vi "Intan_writeDataAcqTimestamp.vi"(3 "hdr fpath":path) -> (1 "timestamp string":string)   [LabVIEW 2020]
panel:
  out "LabVIEW TimeStamp":timestamp
  out "Date Formatted with Milliseconds":string
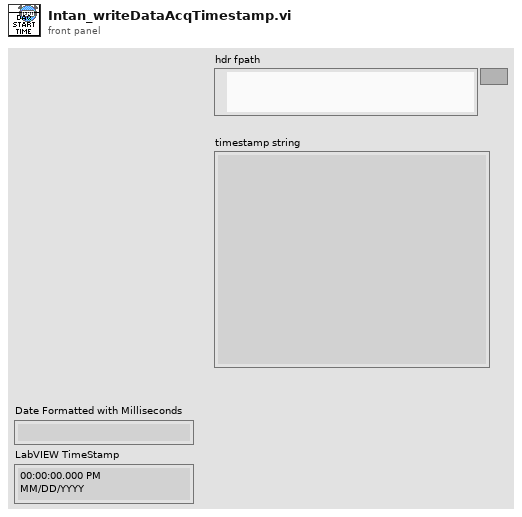
[diagram p1: front panel]
types:
  T1 = enum16{"open", "replace", "create", "open or create", "replace or create", "replace or create with confirmation"}
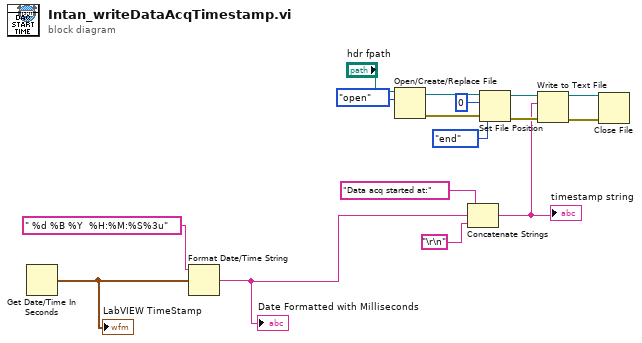
[diagram p0: block diagram]
diagram:
  n1 = Get Date/Time In Seconds() -> (seconds since 1Jan1904=w2:timestamp)
  "LabVIEW TimeStamp" <- w2
  n2 = Format Date/Time String(time format string (%c)=" %d %B %Y  %H:%M:%S%3u", seconds (now)=w2) -> (date/time string=w1:string)  [unwired: 1 in]
  "Date Formatted with Milliseconds" <- w1
  n3 = Open/Create/Replace File(file path (use dialog)="hdr fpath", operation (0:open)=T1."open") -> (refnum out=w12:refnum<file>, error out=w9:errorcluster)  [unwired: 4 in, 1 out]
  n4 = Concatenate Strings("Data acq started at:" ("string"), w1, "\r\n") -> (w6:string)
  "timestamp string" <- w6
  n5 = Set File Position(offset (in bytes) (0)=i64 0, refnum=w12, from (0:start)=enum16{"start", "end", "current"}."end", error in=w9) -> (refnum out=w11:refnum<file>, error out=w10:errorcluster)
  n6 = Write to Text File(file (use dialog)=w11, text=w6, error in=w10) -> (refnum out=w5:refnum<file>, error out=w4:errorcluster)  [unwired: 1 in, 1 out]
  n7 = Close File(refnum=w5, error in=w4) -> ()  [unwired: 2 out]
